vi "obstacleAvoidance.vi"() -> ()   [LabVIEW 2015]
panel:
  in  "stop":bool
  in  "delay (s)":dbl(slide) scale=0.0..0.25
  out "Image":T1(plugin-control)
  out "Image 2":T1(plugin-control)
  in  "Video Sequence Folder Path":path
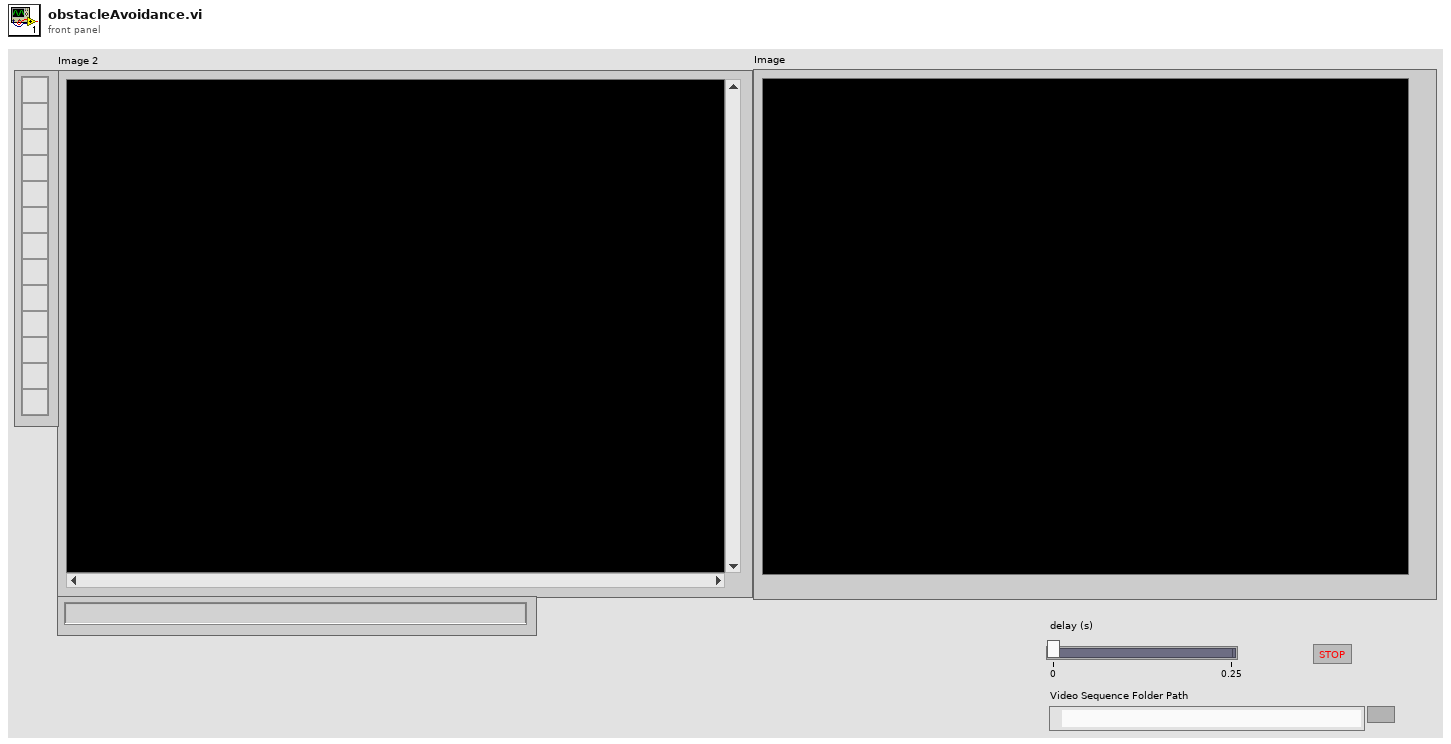
[diagram p1: front panel]
types:
  T1 = typedef "IMAQ Image.ctl" = refnum<image>
  T2 = cluster{"Left":i32, "Top":i32, "Right":i32, "Bottom":i32}
  T3 = typedef "Image Type" = u32
  T4 = cluster{"Global Rectangle":i32[], "Contours":cluster{"Contour Type":u32, "ROI Type":u32, "Points":i32[]}[]}
  T5 = typedef "IMAQ Rectangle" = cluster{"Left":i32, "Top":i32, "Right":i32, "Bottom":i32, "Rotation":dbl}
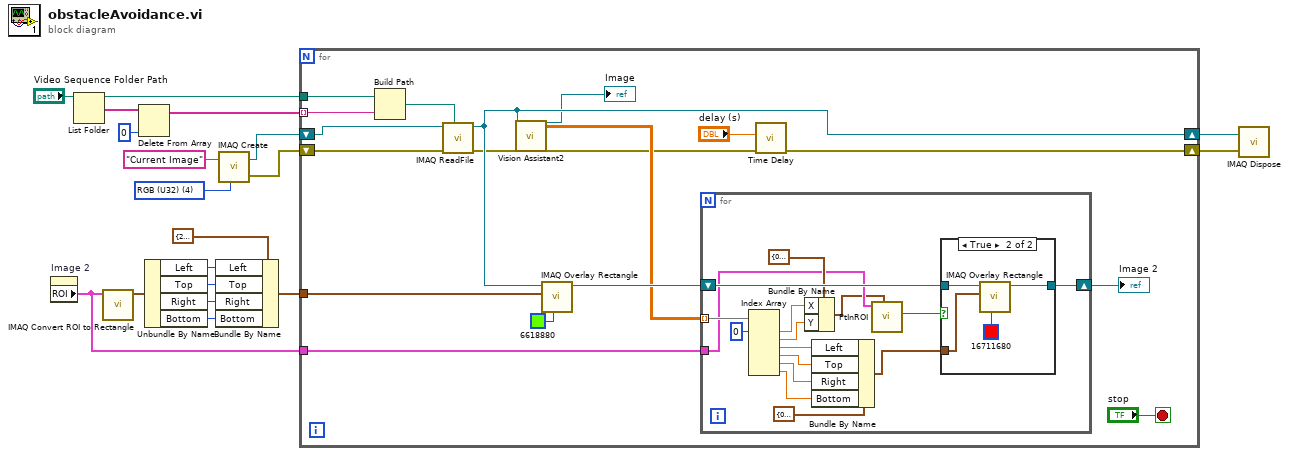
[diagram p0: block diagram]
diagram:
  w14 = T3 4 items=["Grayscale (U8)", "Grayscale (I16)", "Grayscale (SGL)", "Complex (CSG)", "RGB (U32)", "HSL (U32)", "RGB (U64)", "Grayscale (U16)"] ("Image Type")
  n1 = property on="Image 2" class="ImageControl"() -> ("ROI"=w1:T4)  [unwired: 2 in, 2 out]
  n2 = List Folder(path="Video Sequence Folder Path") -> (path out=w16:path, filenames=w19:string[])  [unwired: 1 in, 4 out]
  n3 = call "IMAQ Convert ROI to Rectangle"("ROI Descriptor"=w1) -> ("Rectangle"=w4:T5)  [unwired: 8 in, 1 out]
  n4 = Delete From Array(array=w19, index=0) -> (array with subset deleted=w15:string[])  [unwired: 1 in, 1 out]
  n5 = Unbundle By Name(w4) -> ("Left"=w5:i32, "Top"=w6:i32, "Right"=w7:i32, "Bottom"=w8:i32)
  n6 = Bundle By Name(cluster=T2 {"Left"=237, "Top"=189, "Right"=1028, "Bottom"=546} ("Rectangle"), "Left"=w5, "Top"=w6, "Right"=w7, "Bottom"=w8) -> (w2:T2)
  n7 = call "IMAQ Create"("Image Name"="Current Image", "Image Type"=w14) -> ("New Image"=w12:T1, "error out"=w11:errorcluster)  [unwired: 2 in, 1 out]
  n8 = for {
    tunnel: w16 -> [w36]
    tunnel: w15 -> [w35] mode=indexing
    shift-right: [w24] -> w10
    shift-left: w12 -> [w34]
    shift-right: [w32] -> w9
    shift-left: w11 -> [w33]
    tunnel: w2 -> [w27]
    tunnel: w1 -> [w26]
    stop <- "stop" stop-if-true
    n9 = Build Path(base path=w36, name or relative path=w35) -> (appended path=w37:path)
    n10 = call "IMAQ ReadFile"("File Path"=w37, "error in (no error)"=w33, "Image"=w34) -> ("error out"=w21:errorcluster, "Image Out"=w24:T1)  [unwired: 2 in, 5 out]
    n11 = call "Vision Assistant2"("Image In"=w24, "error in"=w21) -> ("Image Out"=→"Image":T1, "Particle Measurements (Pixels) (Particle Analysis 1)"=w22:dbl[][], "error out"=w20:errorcluster)  [unwired: 23 in]
    n12 = call "IMAQ Overlay Rectangle"("Color"=u32 6618880, "Rectangle"=w27, "Image"=w24) -> ("Image Out"=w29:T1)  [unwired: 7 in, 1 out]
    n13 = for {
      tunnel: w26 -> [w46]
      shift-right: [w52] -> w28
      shift-left: w29 -> [w53]
      tunnel: w22 -> [w50] mode=indexing
      n14 = Index Array(array=w50, index #1=0 ("index")) -> (element #1=w48:dbl, element #2=w47:dbl, element #3=w42:dbl, element #4=w41:dbl, element #5=w40:dbl, element #6=w39:dbl)  [unwired: 5 in]
      n15 = Bundle By Name(cluster=cluster{"X":dbl, "Y":dbl} {"X"=0.0, "Y"=0.0} ("Point"), "X"=w48, "Y"=w47) -> (w44:cluster{"X":dbl, "Y":dbl})
      n16 = Bundle By Name(cluster=T2 {"Left"=0, "Top"=0, "Right"=0, "Bottom"=0} ("Rectangle"), "Left"=w42, "Top"=w41, "Right"=w40, "Bottom"=w39) -> (w38:T2)
      n17 = call "PtInROI.vi"("Point"=w44, "ROI Descriptor In"=w46) -> ("IsInside"=w45:bool)  [unwired: 8 in, 1 out]
      n18 = case shown="True" w45 {
        tunnel: w53 -> [w54 w58]
        tunnel: [w54 w55] -> w52
        tunnel: w38 -> [_ w56]
        frame False {
        }
        frame True {
          n19 = call "IMAQ Overlay Rectangle"("Color"=u32 16711680 ("color(green)"), "Rectangle"=w56, "Image"=w58) -> ("Image Out"=w55:T1)  [unwired: 7 in, 1 out]
        }
      }
    }
    "Image 2" <- w28
    n20 = call "Time Delay"("error in (no error)"=w20, "Delay Time (s)"="delay (s)") -> ("error out"=w32:errorcluster)  [unwired: 9 in]
  }
  n21 = call "IMAQ Dispose"("Image"=w10, "error in (no error)"=w9) -> ()  [unwired: 4 in, 1 out]
